vi "ReadCameraTemperature.vi"(8 "error in (no error)":errorcluster, 11 "Photometrics_CH-250 in":refnum<class "Photometrics_CH-250_Cam.lvclass">) -> (0 "error out":errorcluster, 3 "Photometrics_CH-250 out":refnum<class "Photometrics_CH-250_Cam.lvclass">)   [LabVIEW 2013, in "Photometrics_CH-250_Cam.lvclass"]
uses:
  Photometrics_CH-250_Cam.lvclass
  CameraSessionClass/CS250-CameraHardwareClass.lvclass
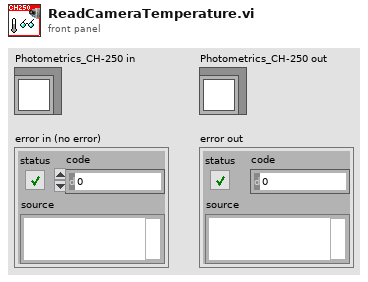
[diagram p1: front panel]
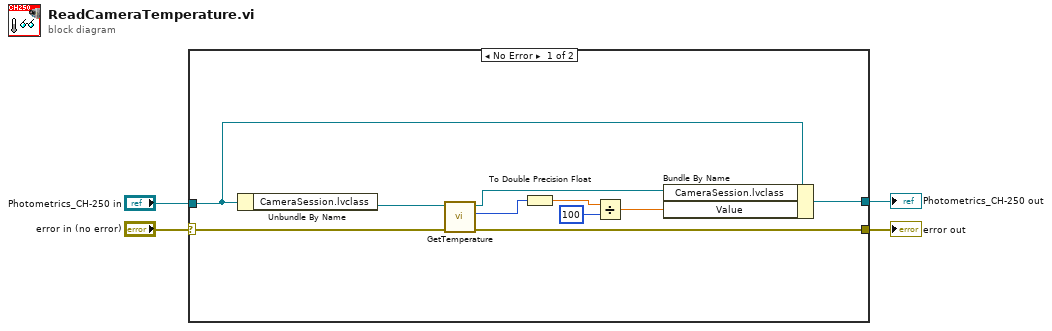
[diagram p0: block diagram]
diagram:
  n1 = case shown="No Error" "error in (no error)" {
    selector: "error in (no error)" -> [w5 w15]
    tunnel: [w14 w16] -> w4
    tunnel: [w13 w15] -> w3
    tunnel: "Photometrics_CH-250 in" -> [w9 w16]
    frame No Error {
      n2 = Unbundle By Name(w9) -> ("CameraSession.lvclass"=w8:refnum<class "CS250-CameraHardwareClass.lvclass">)
      n3 = call-dynamic "GetTemperature.vi"("error in (no error)"=w5, "CameraSession  in"=w8) -> ("error out"=w13:errorcluster, "TReading(degC/100)"=w10:i16, "CameraSession out"=w7:refnum<class "CS250-CameraHardwareClass.lvclass">)  [unwired: 7 in]
      n4 = To Double Precision Float(number=w10) -> (double precision float=w6:dbl)
      n5 = Divide(x=w6, y=i16 100) -> (x/y=w12:dbl)
      n6 = Bundle By Name(cluster=w9, "CameraSession.lvclass"=w7, "Value"=w12) -> (w14:refnum<class "Photometrics_CH-250_Cam.lvclass">)
    }
    frame Error {
    }
  }
  "Photometrics_CH-250 out" <- w4
  "error out" <- w3
